vi "Remove last item from string.vi"(10 "Separator (\\)":string="\\", 11 "String":string) -> (2 "item":string, 3 "String w/o item":string)   [LabVIEW 2013, in "XML Parser.lvclass"]
uses:
  XML Parser.lvclass
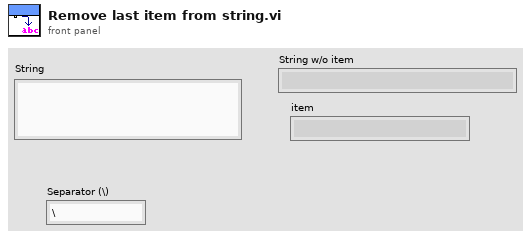
[diagram p1: front panel]
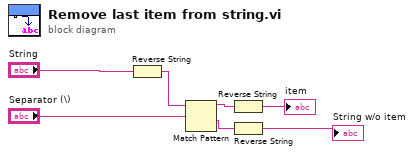
[diagram p0: block diagram]
diagram:
  n1 = Reverse String(1:"String") -> (0:w7:string)
  n2 = Match Pattern(string=w7, regular expression="Separator (\\)") -> (before substring=w6:string, after substring=w2:string)  [unwired: 1 in, 2 out]
  n3 = Reverse String(1:w6) -> (0:→"item":string)
  n4 = Reverse String(1:w2) -> (0:→"String w/o item":string)
